vi "Write Vertical Scroll.vi"(8 "error in (no error)":errorcluster, 10 "Horizontal Scroll":T1 caption="Vertical Scroll", 11 "Panel Object in":refnum<class "Panel Object.lvclass">) -> (0 "error out":errorcluster, 3 "Panel Object out":refnum<class "Panel Object.lvclass">)   [LabVIEW 2015, in "Panel Object.lvclass"]
uses:
  Panel Object.lvclass
  Typedefs/Scrollbar Visibility--Enum.ctl
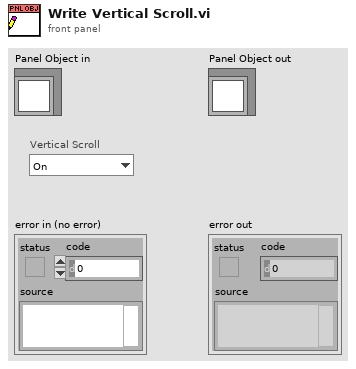
[diagram p1: front panel]
types:
  T1 = typedef "Scrollbar Visibility--Enum.ctl" = enum16{"On", "Off", "Off (Runtime)"}
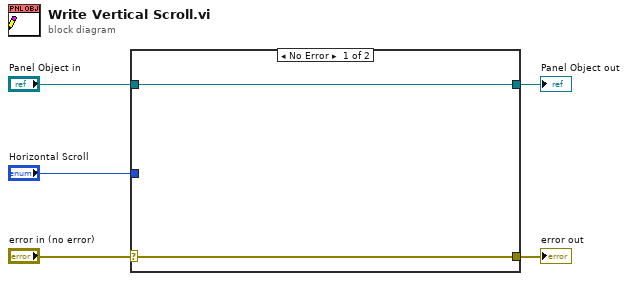
[diagram p0: block diagram]
diagram:
  n1 = case shown="No Error" "error in (no error)" {
    selector: "error in (no error)" -> [w7 w8]
    tunnel: [w7 w8] -> w4
    tunnel: [w6 w9] -> w2
    tunnel: "Panel Object in" -> [w6 w9]
    tunnel: "Horizontal Scroll" -> [_ _]
    frame No Error {
    }
    frame Error {
    }
  }
  "error out" <- w4
  "Panel Object out" <- w2
